vi "action.vi"(0 "HGF_FGV_VisitByName":refnum<class "HGF_FGV_VisitByName.lvclass">, 2 "Objects":refnum<class>[](array[class]), 5 "error in (no error)":errorcluster) -> (14 "dup HGF_FGV_VisitByName":refnum<class "HGF_FGV_VisitByName.lvclass">, 16 "dup Objects":refnum<class>[](array[class]), 19 "error out":errorcluster)   [LabVIEW 2012, in "HGF_FGV.lvlib" / "HGF_FGV_VisitByName.lvclass"]
doc: "Visit selected objects from object array."
uses:
  HGF_FGV_VisitByName.lvclass
  HGF_Base/HGF_Base.lvclass
  HGF_FGV_VisitByName.lvclass/HGF_FGV_VisitByName.ctl
  HGF_FGV_VisitSelection/HGF_FGV_VisitSelection.lvclass
  HGF_Factory/HGF_Factory.lvclass
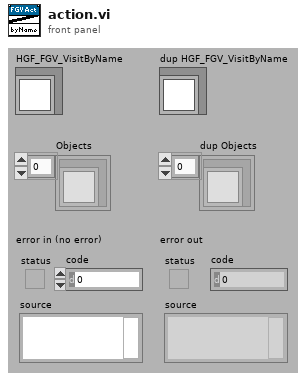
[diagram p1: front panel]
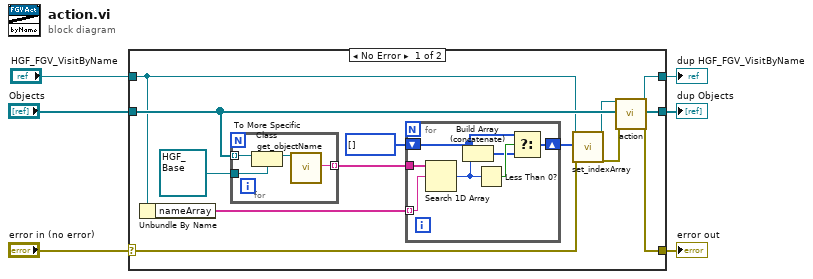
[diagram p0: block diagram]
diagram:
  n1 = case shown="No Error" "error in (no error)" {
    selector: "error in (no error)" -> [w8 w33]
    tunnel: [w12 w33] -> w5
    tunnel: [w15 w32] -> w3
    tunnel: "HGF_FGV_VisitByName" -> [w10 w32]
    tunnel: [w13 w31] -> w2
    tunnel: "Objects" -> [w14 w31]
    frame No Error {
      n2 = Unbundle By Name(w10) -> ("nameArray"=w18:string[])
      n3 = for {
        tunnel: w14 -> [w29] mode=indexing
        tunnel: refnum<class "HGF_Base.lvclass"> refnum ("HGF_BaseClasses.lvlib:HGF_Base.lvclass") -> [w28]
        tunnel: [w27] -> w17 mode=indexing
        n4 = To More Specific Class(target class=w28, reference=w29) -> (specific class reference=w30:refnum<class "HGF_Base.lvclass">)  [unwired: 1 in, 1 out]
        n5 = call "get_objectName.vi"("HGF_Factory"=w30) -> ("objectName"=w27:string)  [unwired: 1 in, 17 out]
      }
      n6 = for {
        tunnel: w18 -> [w25] mode=indexing
        tunnel: w17 -> [w26]
        shift-right: [w20] -> w11
        shift-left: u32[] [] -> [w23]
        n7 = Search 1D Array(1D array=w26, element=w25) -> (index of element=w21:i32)  [unwired: 1 out]
        n8 = Build Array (concatenate)(w23, w21) -> (w22:u32[])
        n9 = Less Than 0?(x=w21) -> (x < 0?=w24:bool)
        n10 = Select(t=w23, s=w24, f=w22) -> (s? t:f=w20:u32[])
      }
      n11 = call "set_indexArray.vi"("HGF_FGV_VisitSelection"=w10, "indexArray"=w11, "error in (no error)"=w8) -> ("dup HGF_FGV_VisitSelection"=w9:refnum<class "HGF_FGV_VisitByName.lvclass">, "error out"=w7:errorcluster)  [unwired: 15 out]
      n12 = call-parent "action.vi"("HGF_FGV_VisitSelection"=w9, "Objects"=w14, "error in (no error)"=w7) -> ("dup HGF_FGV_VisitSelection"=w15:refnum<class "HGF_FGV_VisitByName.lvclass">, "dup Objects"=w13:refnum<class>[], "error out"=w12:errorcluster)  [unwired: 14 out]
    }
    frame Error {
    }
  }
  "error out" <- w5
  "dup HGF_FGV_VisitByName" <- w3
  "dup Objects" <- w2
